vi "Volt to Wave.vi"(1 "Voltage":dbl[unit] min=-0.0745234 max=0.8369266000000001) -> (0 "Retardance":dbl[unit])   [LabVIEW 2009, in "LCD Retarder.lvclass"]
uses:
  LCD Retarder.lvclass
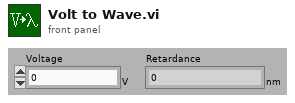
[diagram p1: front panel]
types:
  T1 = cluster{"Wavelength":sgl[unit], "Voltage":sgl[unit]}[]
  T2 = cluster{"Voltage":sgl[unit], "Wavelength":sgl[unit]}
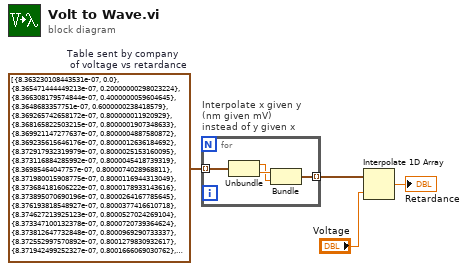
[diagram p0: block diagram]
diagram:
  w4 = T1 [{"Wavelength"=8.36323e-07, "Voltage"=0.0}, {"Wavelength"=8.3654714e-07, "Voltage"=0.2}, {"Wavelength"=8.366308e-07, "Voltage"=0.4}, {"Wavelength"=8.3648683e-07, "Voltage"=0.6}, {"Wavelength"=8.369266e-07, "Voltage"=0.8}, {"Wavelength"=8.368166e-07, "Voltage"=0.8000002}, {"Wavelength"=8.369921e-07, "Voltage"=0.8000005}, {"Wavelength"=8.3692356e-07, "Voltage"=0.80000126}, {"Wavelength"=8.372918e-07, "Voltage"=0.8000025}, {"Wavelength"=8.373117e-07, "Voltage"=0.80000454}, {"Wavelength"=8.3698546e-07, "Voltage"=0.8000074}, {"Wavelength"=8.37198e-07, "Voltage"=0.8000117}, {"Wavelength"=8.373684e-07, "Voltage"=0.8000179}, {"Wavelength"=8.373895e-07, "Voltage"=0.8000264}, {"Wavelength"=8.376194e-07, "Voltage"=0.80003774}, {"Wavelength"=8.374627e-07, "Voltage"=0.8000527}, {"Wavelength"=8.373347e-07, "Voltage"=0.8000721}, {"Wavelength"=8.3738126e-07, "Voltage"=0.8000969}, {"Wavelength"=8.372553e-07, "Voltage"=0.800128}, {"Wavelength"=8.3719425e-07, "Voltage"=0.8001666}, {"Wavelength"=8.3712985e-07, "Voltage"=0.800214}, {"Wavelength"=8.3703804e-07, "Voltage"=0.80027163}, {"Wavelength"=8.371233e-07, "Voltage"=0.8003411}, {"Wavelength"=8.370791e-07, "Voltage"=0.80042404}, {"Wavelength"=8.374333e-07, "Voltage"=0.80052227}, {"Wavelength"=8.37621e-07, "Voltage"=0.800638}, {"Wavelength"=8.374173e-07, "Voltage"=0.8007734}, {"Wavelength"=8.37423e-07, "Voltage"=0.8009308}, {"Wavelength"=8.3697114e-07, "Voltage"=0.80111295}, {"Wavelength"=8.373932e-07, "Voltage"=0.8013225}, {"Wavelength"=8.375728e-07, "Voltage"=0.8015625}, {"Wavelength"=8.375034e-07, "Voltage"=0.80183613}, {"Wavelength"=8.377062e-07, "Voltage"=0.8021468}, {"Wavelength"=8.376599e-07, "Voltage"=0.8024982}, {"Wavelength"=8.375027e-07, "Voltage"=0.8028941}, {"Wavelength"=8.375476e-07, "Voltage"=0.8033387}, {"Wavelength"=8.3769953e-07, "Voltage"=0.8038364}, {"Wavelength"=8.375887e-07, "Voltage"=0.80439174}, {"Wavelength"=8.369123e-07, "Voltage"=0.80500954}, {"Wavelength"=8.364832e-07, "Voltage"=0.8056949}, {"Wavelength"=8.369223e-07, "Voltage"=0.8064534}, {"Wavelength"=8.376672e-07, "Voltage"=0.8072906}, {"Wavelength"=8.37798e-07, "Voltage"=0.8082125}, {"Wavelength"=8.379103e-07, "Voltage"=0.8092255}, {"Wavelength"=8.379108e-07, "Voltage"=0.810336}, {"Wavelength"=8.379115e-07, "Voltage"=0.8115509}, {"Wavelength"=8.3805486e-07, "Voltage"=0.8128775}, {"Wavelength"=8.378885e-07, "Voltage"=0.8143233}, {"Wavelength"=8.37723e-07, "Voltage"=0.8158961}, {"Wavelength"=8.3731896e-07, "Voltage"=0.8176041}, {"Wavelength"=8.36487e-07, "Voltage"=0.81945586}, {"Wavelength"=8.368232e-07, "Voltage"=0.8214603}, {"Wavelength"=8.366337e-07, "Voltage"=0.8236266}, {"Wavelength"=8.370427e-07, "Voltage"=0.8259644}, {"Wavelength"=8.3763507e-07, "Voltage"=0.8284838}, {"Wavelength"=8.376052e-07, "Voltage"=0.8311949}, {"Wavelength"=8.373762e-07, "Voltage"=0.8341088}, {"Wavelength"=8.37485e-07, "Voltage"=0.83723634}, {"Wavelength"=8.3765275e-07, "Voltage"=0.84058917}, {"Wavelength"=8.373148e-07, "Voltage"=0.8441794}, {"Wavelength"=8.3712484e-07, "Voltage"=0.84801924}, {"Wavelength"=8.372684e-07, "Voltage"=0.8521216}, {"Wavelength"=8.373965e-07, "Voltage"=0.85649955}, {"Wavelength"=8.375211e-07, "Voltage"=0.8611669}, {"Wavelength"=8.375448e-07, "Voltage"=0.8661377}, {"Wavelength"=8.3786546e-07, "Voltage"=0.8714266}, {"Wavelength"=8.377302e-07, "Voltage"=0.87704855}, {"Wavelength"=8.3797335e-07, "Voltage"=0.8830189}, {"Wavelength"=8.375698e-07, "Voltage"=0.8893539}, {"Wavelength"=8.377095e-07, "Voltage"=0.8960698}, {"Wavelength"=8.376261e-07, "Voltage"=0.9031836}, {"Wavelength"=8.374067e-07, "Voltage"=0.9107126}, {"Wavelength"=8.3772306e-07, "Voltage"=0.918675}, {"Wavelength"=8.375963e-07, "Voltage"=0.9270889}, {"Wavelength"=8.374703e-07, "Voltage"=0.9359734}, {"Wavelength"=8.3749404e-07, "Voltage"=0.9453481}, {"Wavelength"=8.370354e-07, "Voltage"=0.9552328}, {"Wavelength"=8.3707897e-07, "Voltage"=0.96564806}, {"Wavelength"=8.367532e-07, "Voltage"=0.97661513}, {"Wavelength"=8.363656e-07, "Voltage"=0.98815525}, {"Wavelength"=8.371436e-07, "Voltage"=1.0002911}, {"Wavelength"=8.3630107e-07, "Voltage"=1.0130452}, {"Wavelength"=8.356263e-07, "Voltage"=1.0264407}, {"Wavelength"=8.350644e-07, "Voltage"=1.040502}, {"Wavelength"=8.345527e-07, "Voltage"=1.055253}, {"Wavelength"=8.341678e-07, "Voltage"=1.0707194}, {"Wavelength"=8.340015e-07, "Voltage"=1.0869262}, {"Wavelength"=8.329595e-07, "Voltage"=1.1039004}, {"Wavelength"=8.308729e-07, "Voltage"=1.1216683}, {"Wavelength"=8.3028084e-07, "Voltage"=1.140258}, {"Wavelength"=8.2787324e-07, "Voltage"=1.1596972}, {"Wavelength"=8.249104e-07, "Voltage"=1.1800147}, {"Wavelength"=8.196542e-07, "Voltage"=1.2012403}, {"Wavelength"=8.142827e-07, "Voltage"=1.2234039}, {"Wavelength"=8.070073e-07, "Voltage"=1.2465363}, {"Wavelength"=7.974213e-07, "Voltage"=1.2706689}, {"Wavelength"=7.877812e-07, "Voltage"=1.2958336}, {"Wavelength"=7.768744e-07, "Voltage"=1.3220634}, {"Wavelength"=7.642053e-07, "Voltage"=1.3493917}, {"Wavelength"=7.4888266e-07, "Voltage"=1.3778527}, {"Wavelength"=7.31905e-07, "Voltage"=1.4074811}, {"Wavelength"=7.1349183e-07, "Voltage"=1.4383125}, {"Wavelength"=6.960246e-07, "Voltage"=1.4703833}, {"Wavelength"=6.770439e-07, "Voltage"=1.5037303}, {"Wavelength"=6.569207e-07, "Voltage"=1.5383914}, {"Wavelength"=6.353716e-07, "Voltage"=1.574405}, {"Wavelength"=6.1340086e-07, "Voltage"=1.6118101}, {"Wavelength"=5.918805e-07, "Voltage"=1.6506468}, {"Wavelength"=5.695836e-07, "Voltage"=1.6909559}, {"Wavelength"=5.466619e-07, "Voltage"=1.7327789}, {"Wavelength"=5.2356205e-07, "Voltage"=1.7761579}, {"Wavelength"=5.008738e-07, "Voltage"=1.8211359}, {"Wavelength"=4.776787e-07, "Voltage"=1.8677567}, {"Wavelength"=4.556566e-07, "Voltage"=1.9160651}, {"Wavelength"=4.254029e-07, "Voltage"=1.9661063}, {"Wavelength"=3.878056e-07, "Voltage"=2.071573}, {"Wavelength"=3.668992e-07, "Voltage"=2.1270933}, {"Wavelength"=3.46132e-07, "Voltage"=2.1845362}, {"Wavelength"=3.263368e-07, "Voltage"=2.243951}, {"Wavelength"=3.073979e-07, "Voltage"=2.3053887}, {"Wavelength"=2.8899788e-07, "Voltage"=2.3688996}, {"Wavelength"=2.7119958e-07, "Voltage"=2.4345367}, {"Wavelength"=2.5474318e-07, "Voltage"=2.502352}, {"Wavelength"=2.387141e-07, "Voltage"=2.5723999}, {"Wavelength"=2.2334869e-07, "Voltage"=2.6447349}, {"Wavelength"=2.0895399e-07, "Voltage"=2.7194126}, {"Wavelength"=1.9528301e-07, "Voltage"=2.7964892}, {"Wavelength"=1.8229319e-07, "Voltage"=2.8760226}, {"Wavelength"=1.701385e-07, "Voltage"=2.9580703}, {"Wavelength"=1.585092e-07, "Voltage"=3.042692}, {"Wavelength"=1.4771139e-07, "Voltage"=3.1299477}, {"Wavelength"=1.372768e-07, "Voltage"=3.2198982}, {"Wavelength"=1.274195e-07, "Voltage"=3.3126056}, {"Wavelength"=1.18426e-07, "Voltage"=3.408133}, {"Wavelength"=1.09792296e-07, "Voltage"=3.5065439}, {"Wavelength"=1.018034e-07, "Voltage"=3.6079032}, {"Wavelength"=9.4081706e-08, "Voltage"=3.7122772}, {"Wavelength"=8.6930704e-08, "Voltage"=3.8197315}, {"Wavelength"=8.01411e-08, "Voltage"=3.9303348}, {"Wavelength"=7.3562205e-08, "Voltage"=4.044155}, {"Wavelength"=6.72826e-08, "Voltage"=4.1612625}, {"Wavelength"=6.11815e-08, "Voltage"=4.281728}, {"Wavelength"=5.58774e-08, "Voltage"=4.4056225}, {"Wavelength"=5.03585e-08, "Voltage"=4.5330195}, {"Wavelength"=4.52886e-08, "Voltage"=4.663992}, {"Wavelength"=4.0276902e-08, "Voltage"=4.7986155}, {"Wavelength"=3.57691e-08, "Voltage"=4.9369645}, {"Wavelength"=3.14288e-08, "Voltage"=5.0791173}, {"Wavelength"=2.61977e-08, "Voltage"=5.2251515}, {"Wavelength"=2.2381201e-08, "Voltage"=5.375145}, {"Wavelength"=1.75257e-08, "Voltage"=5.5291786}, {"Wavelength"=1.3356201e-08, "Voltage"=5.6873336}, {"Wavelength"=8.9312e-09, "Voltage"=5.849692}, {"Wavelength"=6.1170997e-09, "Voltage"=6.0163364}, {"Wavelength"=2.7457e-09, "Voltage"=6.187352}, {"Wavelength"=0.0, "Voltage"=6.362823}, {"Wavelength"=-6.3624e-09, "Voltage"=6.7274823}, {"Wavelength"=-7.2698003e-09, "Voltage"=6.9168463}, {"Wavelength"=-1.2379799e-08, "Voltage"=7.111019}, {"Wavelength"=-1.55156e-08, "Voltage"=7.310092}, {"Wavelength"=-1.73673e-08, "Voltage"=7.514157}, {"Wavelength"=-2.0081e-08, "Voltage"=7.723307}, {"Wavelength"=-2.27045e-08, "Voltage"=7.9376373}, {"Wavelength"=-2.51439e-08, "Voltage"=8.157243}, {"Wavelength"=-2.84332e-08, "Voltage"=8.382221}, {"Wavelength"=-3.08633e-08, "Voltage"=8.61267}, {"Wavelength"=-3.29302e-08, "Voltage"=8.848688}, {"Wavelength"=-3.49179e-08, "Voltage"=9.090377}, {"Wavelength"=-3.66534e-08, "Voltage"=9.337836}, {"Wavelength"=-3.87854e-08, "Voltage"=9.59117}, {"Wavelength"=-4.07057e-08, "Voltage"=9.850481}, {"Wavelength"=-4.2575902e-08, "Voltage"=10.115876}, {"Wavelength"=-4.4192902e-08, "Voltage"=10.387461}, {"Wavelength"=-4.59911e-08, "Voltage"=10.665342}, {"Wavelength"=-4.75694e-08, "Voltage"=10.949632}, {"Wavelength"=-4.9164e-08, "Voltage"=11.240437}, {"Wavelength"=-5.04794e-08, "Voltage"=11.537869}, {"Wavelength"=-5.2011902e-08, "Voltage"=11.842042}, {"Wavelength"=-5.3556597e-08, "Voltage"=12.153069}, {"Wavelength"=-5.48978e-08, "Voltage"=12.4710655}, {"Wavelength"=-5.62867e-08, "Voltage"=12.796148}, {"Wavelength"=-5.74831e-08, "Voltage"=13.128434}, {"Wavelength"=-5.87499e-08, "Voltage"=13.468044}, {"Wavelength"=-5.99905e-08, "Voltage"=13.815097}, {"Wavelength"=-6.1204396e-08, "Voltage"=14.169714}, {"Wavelength"=-6.22968e-08, "Voltage"=14.53202}, {"Wavelength"=-6.33501e-08, "Voltage"=14.902137}, {"Wavelength"=-6.452839e-08, "Voltage"=15.280192}, {"Wavelength"=-6.5550005e-08, "Voltage"=15.666313}, {"Wavelength"=-6.65714e-08, "Voltage"=16.060627}, {"Wavelength"=-6.74981e-08, "Voltage"=16.463264}, {"Wavelength"=-6.8468495e-08, "Voltage"=16.874353}, {"Wavelength"=-6.9371595e-08, "Voltage"=17.294031}, {"Wavelength"=-7.0283996e-08, "Voltage"=17.722427}, {"Wavelength"=-7.11298e-08, "Voltage"=18.159681}, {"Wavelength"=-7.20201e-08, "Voltage"=18.605927}, {"Wavelength"=-7.2892895e-08, "Voltage"=19.0613}, {"Wavelength"=-7.372989e-08, "Voltage"=19.525946}, {"Wavelength"=-7.45234e-08, "Voltage"=20.0}]  # Table sent by company  of voltage vs retardance
  n1 = for "Interpolate x given y\n(nm given mV)\ninstead of y given x" {
    tunnel: w4 -> [w8] mode=indexing
    tunnel: [w5] -> w3 mode=indexing
    n2 = Unbundle(w8) -> ("Wavelength"=w6:sgl[unit], "Voltage"=w7:sgl[unit])
    n3 = Bundle("Voltage"=w7, "Wavelength"=w6) -> (w5:T2)  [unwired: 1 out]
  }
  n4 = Interpolate 1D Array(1:"Voltage", 2:w3) -> (0:→"Retardance":sgl[unit])
